vi "ex3.vi"() -> ()   [LabVIEW 2022 SP3]
uses:
  #typedef_ex3_states.ctl
panel:
  in  "Draught level [ml]":dbl(slide) scale=0.0..50.0
  in  "Drink Beer":bool
  in  "No More drinking":bool
  out "Beer":dbl(slide) scale=0.0..500.0
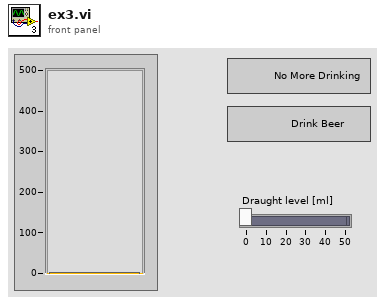
[diagram p1: front panel]
types:
  T1 = typedef "#typedef_ex3_states.ctl" = enum16{"Initialization", "Less than 50", "Refresh GUI", "Drink Beer ", "No More Drinking", "Error Handler", "Idle"}
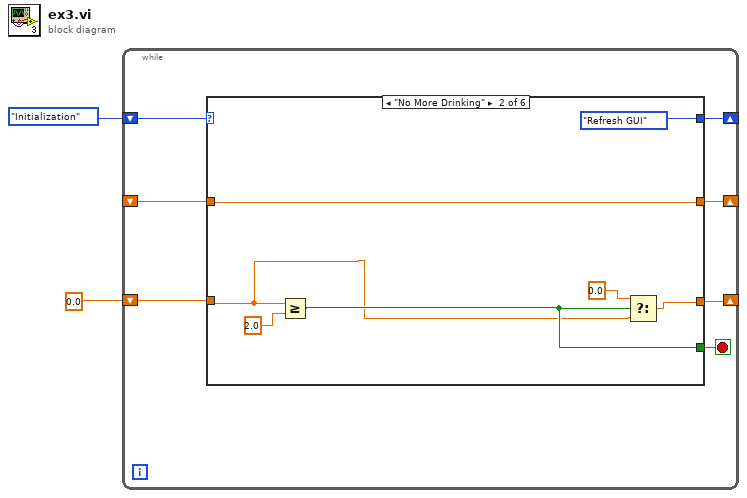
[diagram p0: block diagram]
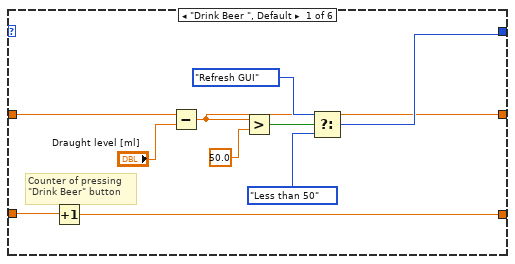
[diagram p2: hidden frame]
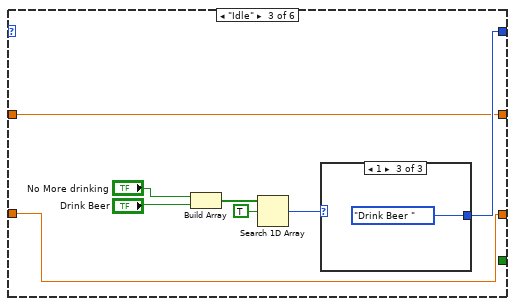
[diagram p3: hidden frame]
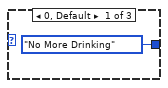
[diagram p4: hidden frame]
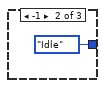
[diagram p5: hidden frame]
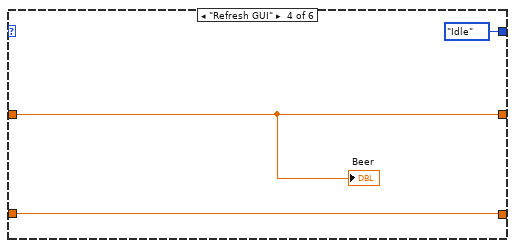
[diagram p6: hidden frame]
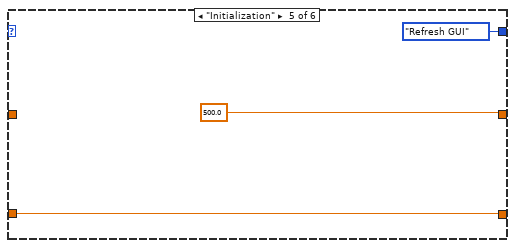
[diagram p7: hidden frame]
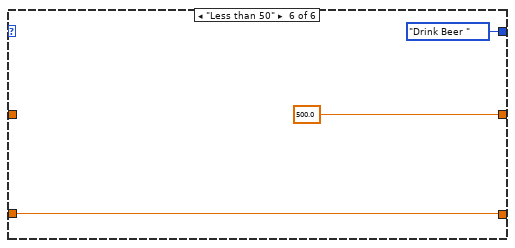
[diagram p8: hidden frame]
diagram:
  n1 = while {
    shift-right: [w7] -> _
    shift-left: _ -> [w8]
    shift-right: [w6] -> _
    shift-left: #typedef_ex3_states."Initialization" ("Enum") -> [w9]
    shift-right: [w4] -> _
    shift-left: 0.0 ("y") -> [w5]
    stop <- w3 stop-if-true
    n2 = case shown="\"No More Drinking\"" w9 {
      tunnel: w8 -> [w19 w26 w28 w40 _ _]
      tunnel: [w12 w26 w28 w40 500.0 ("Beer") 500.0] -> w7
      tunnel: [w13 #typedef_ex3_states."Refresh GUI" ("Enum") w29 #typedef_ex3_states."Idle" ("Enum") #typedef_ex3_states."Refresh GUI" ("Enum") #typedef_ex3_states."Drink Beer " ("Enum")] -> w6
      tunnel: w5 -> [w11 w21 w27 w38 w41 w44]
      tunnel: [w10 w20 w27 w38 w41 w44] -> w4
      tunnel: [_ w23 _ _ _ _] -> w3
      frame "Drink Beer ", Default {
        # "Counter of pressing \n\"Drink Beer\" button"
        n3 = Increment(x=w11) -> (x+1=w10:dbl)
        n4 = Subtract(x=w19, y="Draught level [ml]") -> (x-y=w12:dbl)
        n5 = Greater?(x=w12, y=50.0) -> (0:w16:bool)
        n6 = Select(t=#typedef_ex3_states."Refresh GUI" ("Enum"), s=w16, f=#typedef_ex3_states."Less than 50" ("Enum")) -> (s? t:f=w13:T1)
      }
      frame "No More Drinking" {
        n7 = Greater Or Equal?(x=w21, y=2.0) -> (x >= y?=w23:bool)
        n8 = Select(t=0.0, s=w23, f=w21) -> (s? t:f=w20:dbl)
      }
      frame "Idle" {
        n9 = Build Array("No More drinking", "Drink Beer") -> (w32:bool[])
        n10 = Search 1D Array(1D array=w32, element=TRUE) -> (index of element=w30:i32)  [unwired: 1 in]
        n11 = case shown="1" w30 {
          tunnel: [#typedef_ex3_states."No More Drinking" ("Enum") #typedef_ex3_states."Idle" ("Enum") #typedef_ex3_states."Drink Beer " ("Enum")] -> w29
          frame 0, Default {
          }
          frame -1 {
          }
          frame 1 {
          }
        }
      }
      frame "Refresh GUI" {
        "Beer" <- w40
      }
      frame "Initialization" {
      }
      frame "Less than 50" {
      }
    }
  }
